vi "tcs shm accept Command standby LV.vi"(8 "error in (no error)":errorcluster, 11 "command_standby_Ctl":cluster{"state":u8}) -> (0 "error out":errorcluster, 2 "function return":i32, 3 "command_standby_Ctl out":cluster{"state":u8})   [LabVIEW 2016, in "SALLV_tcs.lvlib"]
doc: "int tcs_shm_acceptCommand_standbyLV(tcs_command_standbyLV *command_standby_Ctl );"
uses:
  SALLV_tcs.lvlib
  SALLV_tcs.so
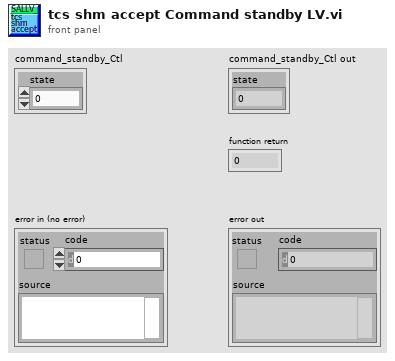
[diagram p1: front panel]
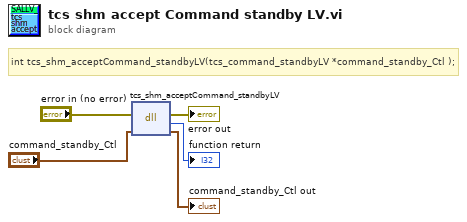
[diagram p0: block diagram]
diagram:
  # "int tcs_shm_acceptCommand_standbyLV(tcs_command_standbyLV *command_standby_Ctl );"
  n1 = dll-call lib="home/plotz/SALLV_tcs/SALLV_tcs.*" fn="tcs_shm_acceptCommand_standbyLV"(error in="error in (no error)", "command_standby_Ctl"="command_standby_Ctl") -> (error out=→"error out":errorcluster, →"function return":i32, "command_standby_Ctl"=→"command_standby_Ctl out":cluster{"state":u8})  [unwired: 2 in, 1 out]
